vi "PAN_TCPSERVER_QueueCmd.vi"(6 "timeout in ms (-1)":i32=10000, 7 "ID":string, 8 "error in (no error)":errorcluster, 9 "response queue":refnum<queue>, 10 "command":string, 11 "queue in":refnum<queue>) -> (0 "error out":errorcluster, 2 "response":string)   [LabVIEW 2016]
uses:
  private/vis/PAN_TCPSERVER_MsgStruct.ctl
panel:
  in  "ResponseStruct":T1
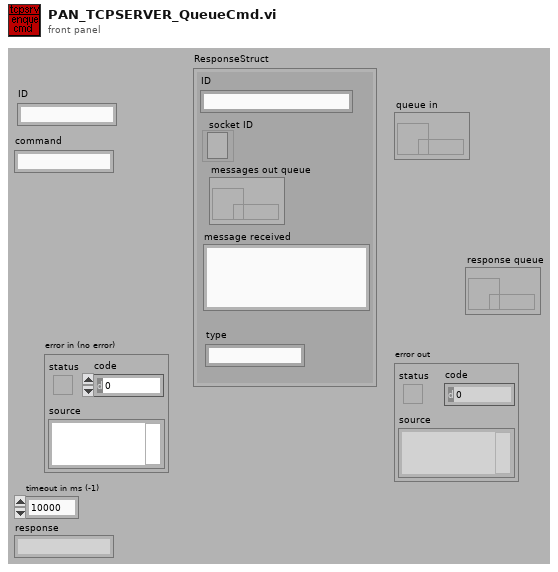
[diagram p1: front panel]
types:
  T1 = typedef "PAN_TCPSERVER_MsgStruct.ctl" = cluster{"ID":string, "socket ID":refnum<k5>, "messages out queue":refnum<queue>, "message received":string, "type":string}
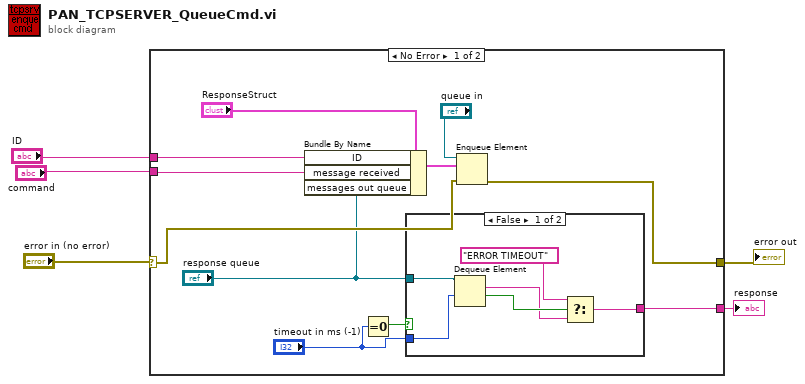
[diagram p0: block diagram]
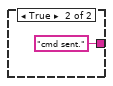
[diagram p2: hidden frame]
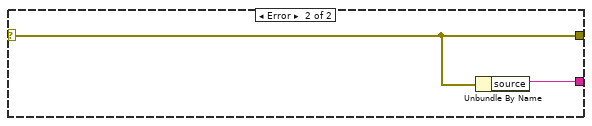
[diagram p3: hidden frame]
diagram:
  n1 = case shown="No Error" "error in (no error)" {
    selector: "error in (no error)" -> [w10 w25]
    tunnel: "ID" -> [w15 _]
    tunnel: "command" -> [w14 _]
    tunnel: [w9 w25] -> w2
    tunnel: [w11 w24] -> w1
    frame No Error {
      n2 = Bundle By Name(cluster="ResponseStruct", "ID"=w15, "message received"=w14, "messages out queue"="response queue") -> (w12:T1)
      n3 = Equal To 0?(x="timeout in ms (-1)") -> (x = 0?=w6:bool)
      n4 = case shown="False" w6 {
        tunnel: "response queue" -> [w22 _]
        tunnel: [w18 "cmd sent."] -> w11
        tunnel: "timeout in ms (-1)" -> [w17 _]
        frame False {
          n5 = Dequeue Element(queue=w22, timeout in ms (-1)=w17) -> (element=w20:string, timed out?=w21:bool)  [unwired: 1 in, 2 out]
          n6 = Select(t="ERROR TIMEOUT", s=w21, f=w20) -> (s? t:f=w18:string)
        }
        frame True {
        }
      }
      n7 = Enqueue Element(queue="queue in", element=w12, error in (no error)=w10) -> (error out=w9:errorcluster)  [unwired: 3 out]
    }
    frame Error {
      n8 = Unbundle By Name(w25) -> ("source"=w24:string)
    }
  }
  "error out" <- w2
  "response" <- w1
